vi "get_image.vi"(8 "error in (no error)":errorcluster, 11 "reference":refnum<k24>) -> (0 "error out":errorcluster, 3 "Array":u8[][](array[numeric]))   [LabVIEW 2014]
uses:
  C:/Program Files (x86)/National Instruments/LabVIEW 2014/instr.lib/IDS/ueye.NET/uEyeDotNet.dll
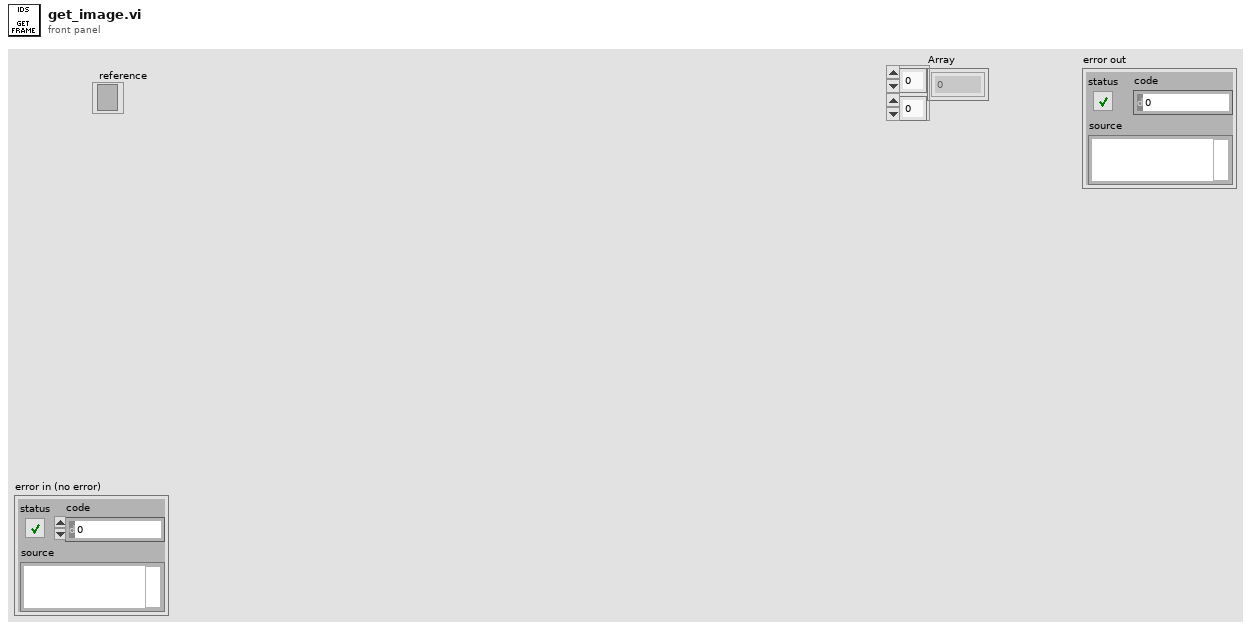
[diagram p1: front panel]
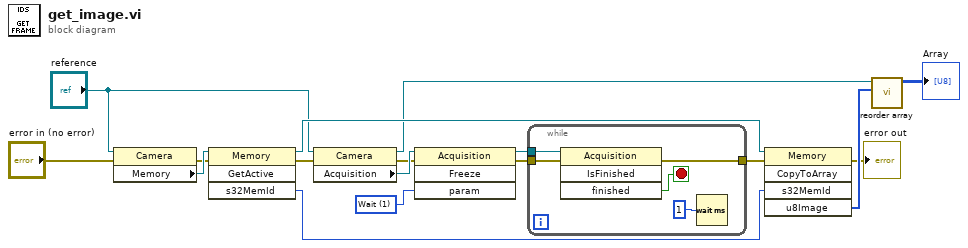
[diagram p0: block diagram]
diagram:
  w12 = 1 items=["DontWait"=0, "Wait"=1, "Force"=16384] ("param")
  n1 = property class="Camera"(reference="reference", error in="error in (no error)") -> (error out=w3:errorcluster, "Memory"=w4:refnum<k24>)  [unwired: 1 out]
  n2 = invoke class="Memory" method="GetActive"(reference=w4, error in=w3) -> (reference out=w16:refnum<k24>, error out=w11:errorcluster, "s32MemId"=w15:i32)  [unwired: 2 in, 1 out]
  n3 = property class="Camera"(reference="reference", error in=w11) -> (reference out=w8:refnum<k24>, error out=w10:errorcluster, "Acquisition"=w17:refnum<k24>)
  n4 = invoke class="Acquisition" method="Freeze"(reference=w17, error in=w10, "param"=w12) -> (reference out=w14:refnum<k24>, error out=w13:errorcluster)  [unwired: 1 in, 2 out]
  n5 = while {
    tunnel: w14 -> [w22]
    tunnel: w13 -> [w21]
    tunnel: [w19] -> w9
    stop <- w20 stop-if-true
    n6 = invoke class="Acquisition" method="IsFinished"(reference=w22, error in=w21) -> (error out=w19:errorcluster, "finished"=w20:bool)  [unwired: 2 in, 2 out]
    n7 = Wait (ms)(milliseconds to wait=u32 1) -> ()  [unwired: 1 out]
  }
  n8 = invoke class="Memory" method="CopyToArray"(reference=w16, error in=w9, "s32MemId"=w15) -> (error out=→"error out":errorcluster, "u8Image"=w7:u8[])  [unwired: 2 in, 3 out]
  n9 = call "reorder array.vi"("InArray"=w7, ".NET (Reference)"=w8) -> ("Array"=→"Array":u8[][])  [unwired: 8 in, 1 out]
